vi "Terminate VI Reference.vi"(8 "error in (no error)":errorcluster, 11 "Reference In":refnum<vi>) -> (0 "error out":errorcluster)   [LabVIEW 2022 SP3]
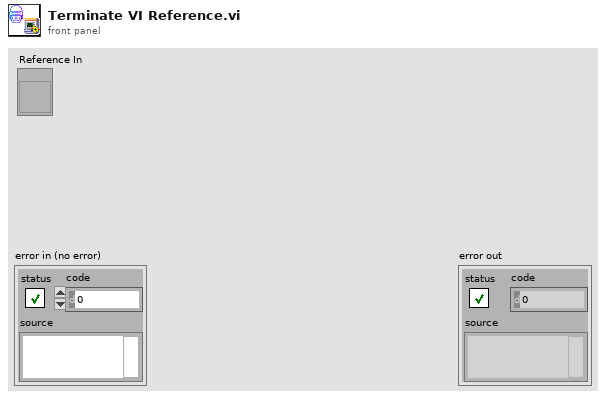
[diagram p1: front panel]
types:
  T1 = enum32{"Bad", "Idle", "Run top level", "Running"}
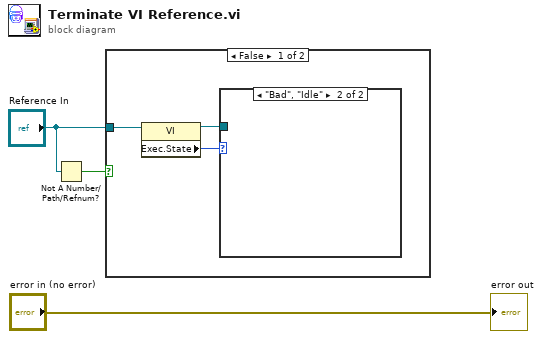
[diagram p0: block diagram]
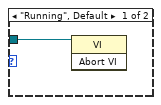
[diagram p2: hidden frame]
diagram:
  n1 = Not A Number/Path/Refnum?(number/path/refnum="Reference In") -> (NaN/Path/Refnum?=w1:bool)
  n2 = case shown="False" w1 {
    tunnel: "Reference In" -> [w4 _]
    frame False {
      n3 = property class="VI"(reference=w4) -> (reference out=w6:refnum<vi>, "Exec.State"=w5:T1)  [unwired: 1 in, 1 out]
      n4 = case shown="\"Bad\", \"Idle\"" w5 {
        tunnel: w6 -> [w7 _]
        frame "Running", Default {
          n5 = invoke class="VI" method="Abort VI"(reference=w7) -> ()  [unwired: 2 in, 3 out]
        }
        frame "Bad", "Idle" {
        }
      }
    }
    frame True {
    }
  }
  "error out" <- "error in (no error)"
